vi "USB2XXX_LINEX_UDSTest.vi"() -> ()   [LabVIEW 2010]
panel:
  out "pLINGetMsg":T1(array[cluster])
  in  "pCanGetMsg":T2
  out "pUDSAddr out 2":T3
  in  "pUDSAddr":T3={"ReqID"=60, "ResID"=61, "NAD"=1, "CheckType"=0, "STmin"=5} {"ReqID" format="%x"; "ResID" format="%x"}
  out "pUDSAddr out":T3
  out "function return":i32
  in  "stop":bool
  out "Readed Data Num":i32
  out "Read Data(Hex)":string
  in  "Write Data(Hex)":string="11 22 33 44 55 66 77 88"
  in  "BaudRate":u32=19200
  in  "Channel Index":u8(ring) items=["LIN1", "LIN2"]
  in  "Device Index":i32(ring) items=["0", "1", "2", "3", "4", "5"]
  # "波特率一定要设置，否则程序可能出错"
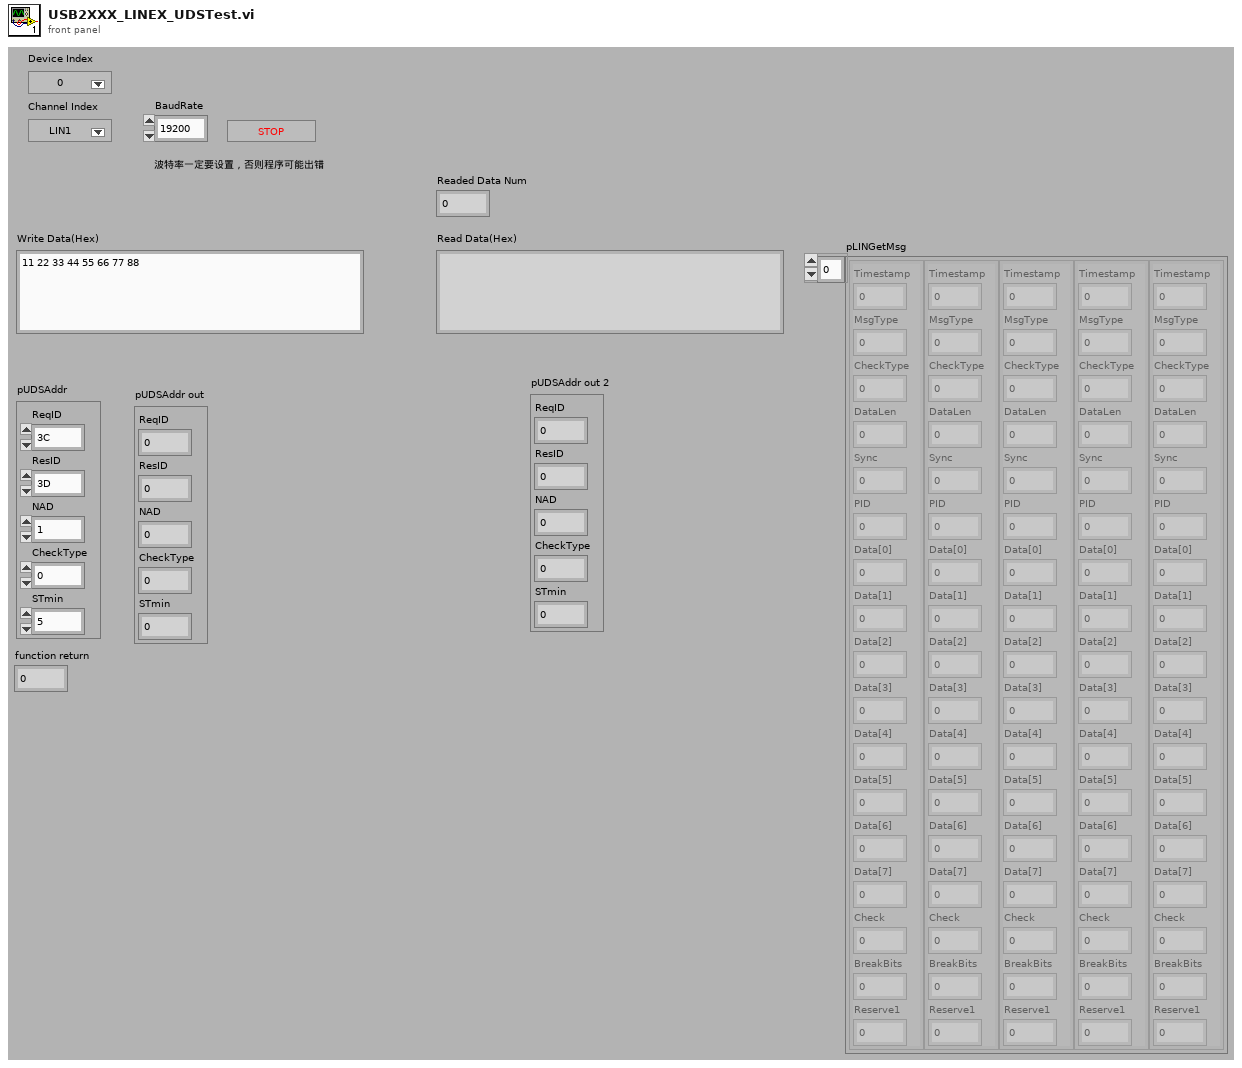
[diagram p1: front panel]
types:
  T1 = cluster{"Timestamp":u32, "MsgType":u8, "CheckType":u8, "DataLen":u8, "Sync":u8, "PID":u8, "Data[0]":u8, "Data[1]":u8, "Data[2]":u8, "Data[3]":u8, "Data[4]":u8, "Data[5]":u8, "Data[6]":u8, "Data[7]":u8, "Check":u8, "BreakBits":u8, "Reserve1":u8}[]
  T2 = cluster{"Timestamp":u32, "MsgType":u8, "CheckType":u8, "DataLen":u8, "Sync":u8, "PID":u8, "Data[0]":u8, "Data[1]":u8, "Data[2]":u8, "Data[3]":u8, "Data[4]":u8, "Data[5]":u8, "Data[6]":u8, "Data[7]":u8, "Check":u8, "BreakBits":u8, "Reserve1":u8}
  T3 = cluster{"ReqID":u8, "ResID":u8, "NAD":u8, "CheckType":u8, "STmin":u8}
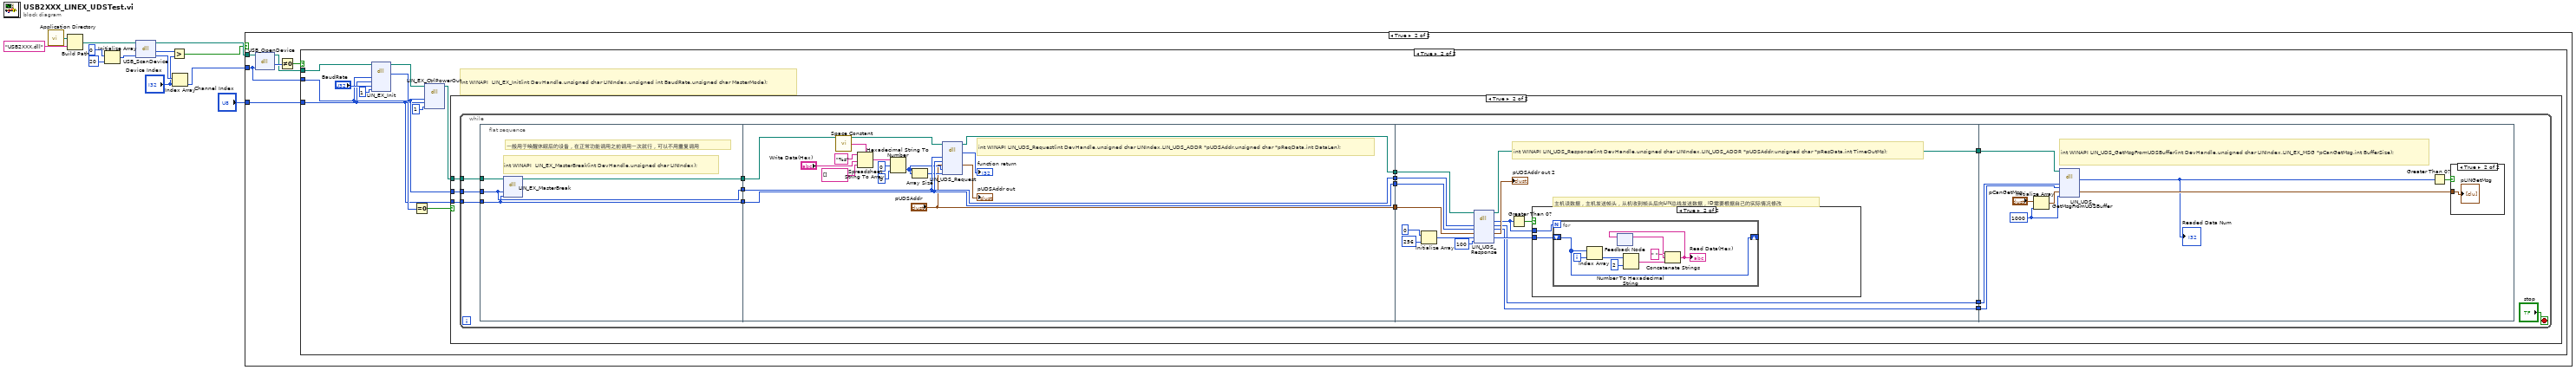
[diagram p0: block diagram]
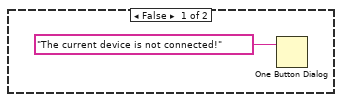
[diagram p2: hidden frame]
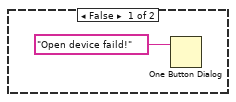
[diagram p3: hidden frame]
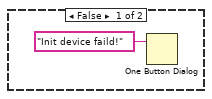
[diagram p4: hidden frame]
diagram:
  n1 = call <vilib>:"Application Directory.vi"() -> ("Application Directory"=w5:path)
  n2 = Build Path(base path=w5, name or relative path="USB2XXX.dll") -> (appended path=w4:path)
  n3 = Initialize Array(0, 20 ("dimension size")) -> (w11:i32[])
  n4 = dll-call lib="E:/OtherWork/STM32/USB2XXX_Example/examples/Labview/PublicFiles/USB2XXX.dll" fn="USB_ScanDevice"(path in=w4, "pDevNum"=w11) -> (path out=w9:path, "return type"=w3:i32, "pDevNum"=w10:i32[])  [unwired: 2 in, 1 out]
  n5 = Greater?(x=w3, y="Device Index") -> (0:w1:bool)
  n6 = Index Array(array=w10, index="Device Index") -> (element=w8:i32)
  n7 = case shown="True" w1 {
    tunnel: w9 -> [_ w20]
    tunnel: w8 -> [_ w16]
    tunnel: "Channel Index" -> [_ w15]
    frame False {
      n8 = One Button Dialog(message="The current device is not connected!") -> ()  [unwired: 1 in, 1 out]
    }
    frame True {
      n9 = dll-call lib="E:/OtherWork/STM32/USB2XXX_Example/examples/Labview/PublicFiles/USB2XXX.dll" fn="USB_OpenDevice"(path in=w20, "DevIndex"=w16) -> (path out=w17:path, "return type"=w19:u8)  [unwired: 3 in, 1 out]
      n10 = Not Equal To 0?(x=w19) -> (x != 0?=w18:bool)
      n11 = case shown="True" w18 {
        tunnel: w17 -> [_ w29]
        tunnel: w16 -> [_ w24]
        tunnel: w15 -> [_ w22]
        frame False {
          n12 = One Button Dialog(message="Open device faild!") -> ()  [unwired: 1 in, 1 out]
        }
        frame True {
          # "int WINAPI  LIN_EX_Init(int DevHandle,unsigned char LINIndex,unsigned int BaudRate,unsigned char MasterMode);"
          n13 = dll-call lib="E:/OtherWork/STM32/USB2XXX_Example/examples/Labview/PublicFiles/USB2XXX.dll" fn="LIN_EX_Init"(path in=w29, "DevHandle"=w24, "LINIndex"=w22, "BaudRate"="BaudRate", "MasterMode"=u8 1) -> (path out=w26:path, "return type"=w28:i32)  [unwired: 6 in, 1 out]
          n14 = Equal To 0?(x=w28) -> (x = 0?=w27:bool)
          n15 = dll-call lib="E:/Projects/USB2XXX/trunk/USB2XXX/USB2XXX/vs2010/Release/USB2XXX.*" fn="LIN_EX_CtrlPowerOut"(path in=w26, "DevHandle"=w24, "LINIndex"=w22, "VbatValue"=u8 1 ("State")) -> (path out=w25:path)  [unwired: 6 in, 1 out]
          n16 = case shown="True" w27 {
            tunnel: w25 -> [_ w35]
            tunnel: w24 -> [_ w34]
            tunnel: w22 -> [_ w33]
            frame False {
              n17 = One Button Dialog(message="Init device faild!") -> ()  [unwired: 1 in, 1 out]
            }
            frame True {
              n18 = while {
                tunnel: w35 -> [w47]
                tunnel: w34 -> [w46]
                tunnel: w33 -> [w45]
                stop <- "stop" stop-if-true
                n19 = flat-sequence {
                  tunnel: w47 -> [w53]
                  tunnel: w46 -> [w51]
                  tunnel: w45 -> [w50]
                  tunnel: [w50] -> w43
                  tunnel: [w51] -> w42
                  tunnel: [w52] -> w41
                  tunnel: [w60] -> w49
                  tunnel: [w59] -> w48
                  tunnel: w43 -> [w59]
                  tunnel: w42 -> [w60]
                  tunnel: w41 -> [w55]
                  tunnel: ["pUDSAddr"] -> w40
                  tunnel: [w54] -> w39
                  tunnel: w49 -> [w79]
                  tunnel: w48 -> [w78]
                  tunnel: w40 -> [w74]
                  tunnel: w39 -> [w73]
                  tunnel: [w72] -> w38
                  tunnel: [w71] -> w37
                  tunnel: [w70] -> w36
                  tunnel: w38 -> [w103]
                  tunnel: w37 -> [w102]
                  tunnel: w36 -> [w101]
                  frame #0 {
                    # "一般用于唤醒休眠后的设备，在正常功能调用之前调用一次就行，可以不用重复调用"
                    # "int WINAPI  LIN_EX_MasterBreak(int DevHandle,unsigned char LINIndex);"
                    n20 = dll-call lib="E:/Projects/USB2XXX/trunk/USB2XXX/USB2XXX/vs2010/Release/USB2XXX.*" fn="LIN_EX_MasterBreak"(path in=w53, "DevHandle"=w51, "LINIndex"=w50) -> (path out=w52:path)  [unwired: 5 in, 1 out]
                  }
                  frame #1 {
                    # "int WINAPI LIN_UDS_Request(int DevHandle,unsigned char LINIndex,LIN_UDS_ADDR *pUDSAddr,unsigned char *pReqData,int DataLen);"
                    n21 = call <vilib>:"Space Constant.vi"() -> ("String"=w65:string)
                    n22 = Spreadsheet String To Array(delimiter (Tab)=w65, format string="%s", spreadsheet string="Write Data(Hex)", array type (2D Dbl)=string[] []) -> (array=w68:string[])
                    n23 = Hexadecimal String To Number(string=w68, offset=0, default (0uL)=u8 0 ("default (0 U32)")) -> (number=w57:u8[])  [unwired: 1 out]
                    n24 = Array Size(array=w57) -> (size(s)=w58:i32)
                    n25 = dll-call lib="E:/OtherWork/STM32/USB2XXX/trunk/USB2XXX/USB2XXX/vs2010/Release/USB2XXX.*" fn="LIN_UDS_Request"(path in=w55, "DevHandle"=w60, "LINIndex"=w59, "pUDSAddr"="pUDSAddr", "pReqData"=w57, "DataLen"=w58) -> (path out=w54:path, "return type"=→"function return":i32, "pUDSAddr"=→"pUDSAddr out":T3)  [unwired: 6 in, 1 out]
                  }
                  frame #2 {
                    # "int WINAPI LIN_UDS_Response(int DevHandle,unsigned char LINIndex,LIN_UDS_ADDR *pUDSAddr,unsigned char *pResData,int TimeOutMs);"
                    # "主机读数据，主机发送帧头，从机收到帧头后向LIN总线发送数据，ID需要根据自己的实际情况修改"
                    n26 = Initialize Array(u8 0 ("element"), 256 ("dimension size")) -> (w77:u8[])
                    n27 = dll-call lib="E:/OtherWork/STM32/USB2XXX/trunk/USB2XXX/USB2XXX/vs2010/Release/USB2XXX.*" fn="LIN_UDS_Response"(path in=w73, "DevHandle"=w79, "LINIndex"=w78, "pUDSAddr"=w74, "pResData"=w77, "TimeOutMs"=100) -> (path out=w72:path, "return type"=w75:i32, "DevHandle"=w71:i32, "LINIndex"=w70:u8, "pUDSAddr"=→"pUDSAddr out 2":T3, "pResData"=w76:u8[])  [unwired: 3 in, 1 out]
                    n28 = Greater Than 0?(x=w75) -> (x > 0?=w84:bool)
                    n29 = case shown="True" w84 {
                      tunnel: w75 -> [_ w86]
                      tunnel: w76 -> [_ w85]
                      frame False {
                      }
                      frame True {
                        n30 = for {
                          N: w86 -> [_]
                          shift-right: [w87] -> _
                          shift-left: w85 -> [w87]
                          i -> [w94]
                          n31 = Index Array(array=w87, index=w94) -> (element=w93:u8)
                          n32 = feedback #1() -> (w91:string)  [unwired: 1 in]
                          n33 = Number To Hexadecimal String(1:i16 2 ("width (-)"), 2:w93) -> (0:w89:string)
                          n34 = Concatenate Strings(w91, " " ("string"), w89) -> (w88:string)
                          "Read Data(Hex)" <- w88
                          n35 = feedback-in #1(w88) -> ()
                        }
                      }
                    }
                  }
                  frame #3 {
                    w98 = 1000 ("dimension size")
                    # "int WINAPI LIN_UDS_GetMsgFromUDSBuffer(int DevHandle,unsigned char LINIndex,LIN_EX_MSG *pCanGetMsg,int BufferSize);"
                    n36 = Initialize Array("pCanGetMsg", w98) -> (w99:T1)
                    n37 = dll-call lib="E:/Projects/USB2XXX/trunk/USB2XXX/USB2XXX/vs2010/Release/USB2XXX.*" fn="LIN_UDS_GetMsgFromUDSBuffer"(path in=w103, "DevHandle"=w102, "LINIndex"=w101, "pCanGetMsg"=w99, "BufferSize"=w98) -> ("return type"=w95:i32, "pCanGetMsg"=w96:T1)  [unwired: 5 in, 2 out]
                    "Readed Data Num" <- w95
                    n38 = Greater Than 0?(x=w95) -> (x > 0?=w97:bool)
                    n39 = case shown="True" w97 {
                      tunnel: w96 -> [_ w104]
                      frame False {
                      }
                      frame True {
                        "pLINGetMsg" <- w104
                      }
                    }
                  }
                }
              }
            }
          }
        }
      }
    }
  }
